vi "Write.vi"(8 "error in (no error)":errorcluster, 10 "write buffer":string, 11 "Simulated Serial in":refnum<class "Simulated Serial.lvclass">) -> (0 "error out":errorcluster, 2 "return count":u32, 3 "Simulated Serial out":refnum<class "Simulated Serial.lvclass">)   [LabVIEW 2020, in "Simulated Serial.lvclass"]
uses:
  Simulated Serial.lvclass
  Simulated Serial.lvclass/Simulated Serial.ctl
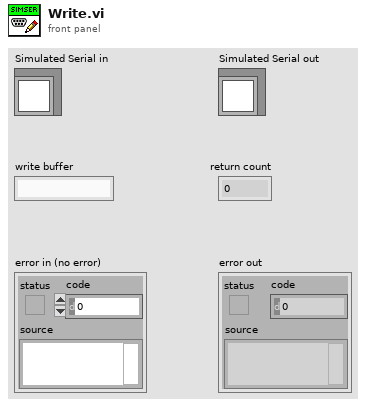
[diagram p1: front panel]
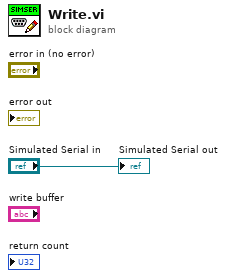
[diagram p0: block diagram]
diagram:
  "Simulated Serial out" <- "Simulated Serial in"
